vi "DRC Send Command_prev.vi"(2 "StringInput":string, 3 "Input":dbl min=0.0 format="%.3f", 4 "Command":T1(ring), 5 "GPIB Address":string) -> (0 "Output":dbl format="%.2f", 1 "Response":string)   [LabVIEW 2019]
panel:
  in  "CHANNEL":bool
  in  "CONTROLLER TYPE":bool
  out "error out":errorcluster
  in  "error in (no error)":errorcluster
  # "setpoint, heater value"
  # "temperature,etc."
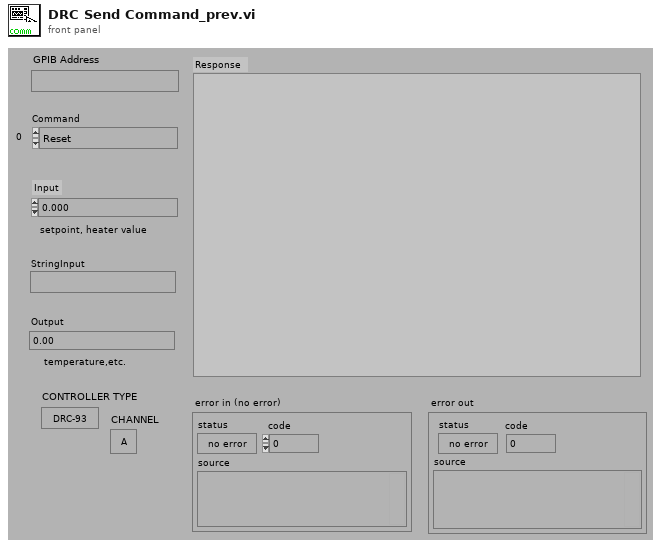
[diagram p1: front panel]
types:
  T1 = enum16{"Reset", "Raw_WriteRead", "ReadTemp", "ReadControl", "WriteSetPoint", "ReadSetPoint", "ManualHeatPwr", "HeaterOff", "SetHeaterScale", "SetProportional(gain)", "SetIntegrate(reset)", "SetDerivative(rate)", "SendCalibration", "ReadCalibration", "SelectCurve", "GetControlInfo", "Change units", "GetDCSP_Reading", "GetPIDR_Reading", "ZeroNonVol_Mem"}
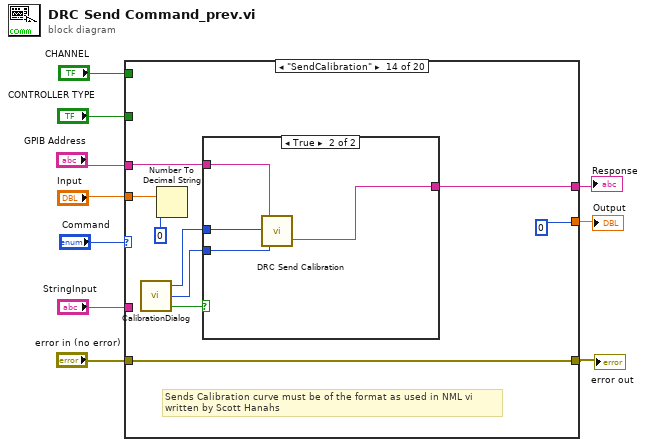
[diagram p0: block diagram]
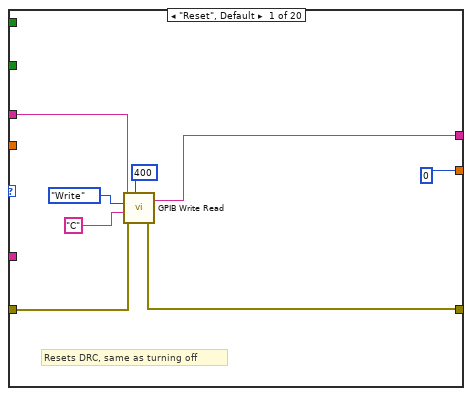
[diagram p2: hidden frame]
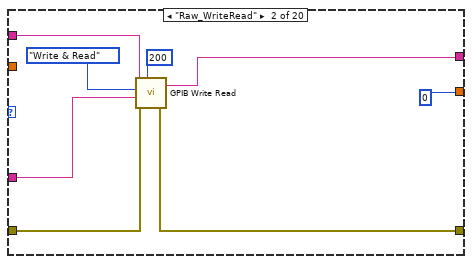
[diagram p3: hidden frame]
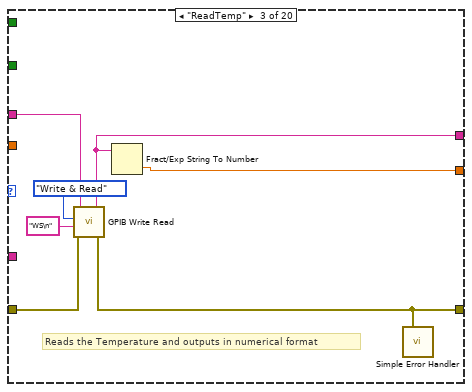
[diagram p4: hidden frame]
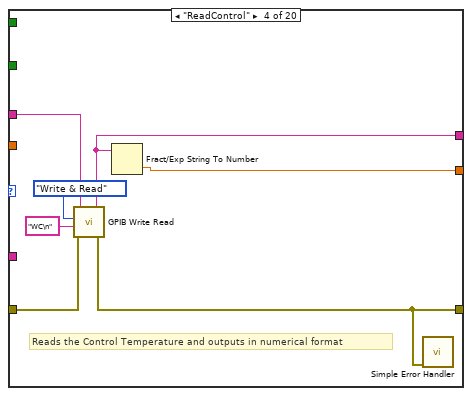
[diagram p5: hidden frame]
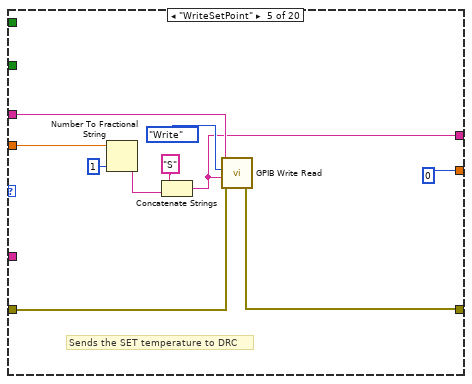
[diagram p6: hidden frame]
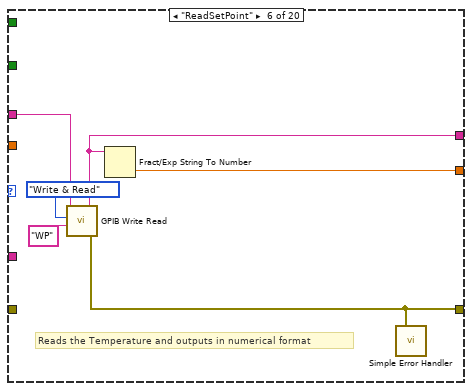
[diagram p7: hidden frame]
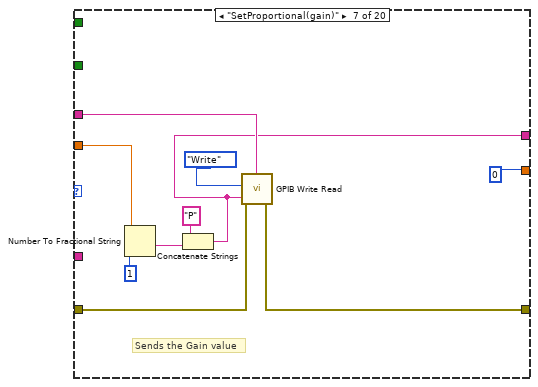
[diagram p8: hidden frame]
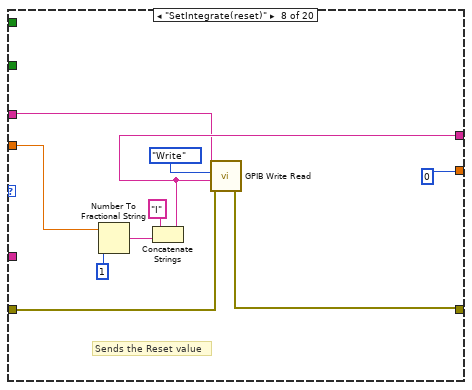
[diagram p9: hidden frame]
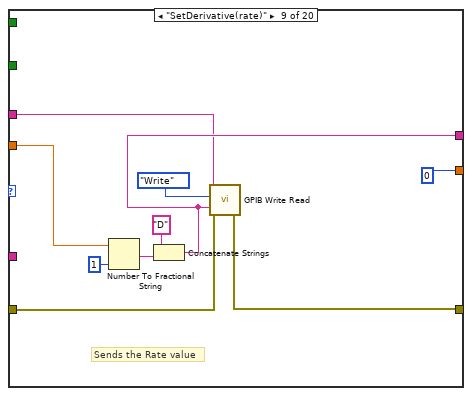
[diagram p10: hidden frame]
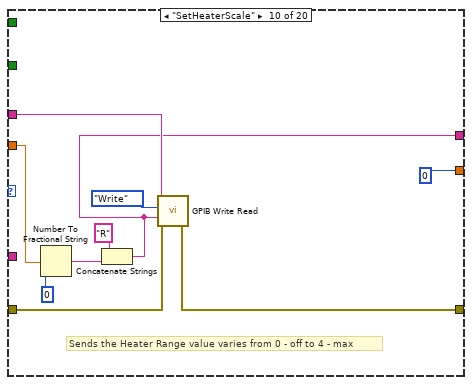
[diagram p11: hidden frame]
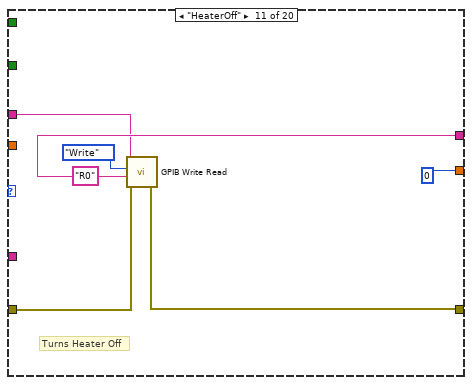
[diagram p12: hidden frame]
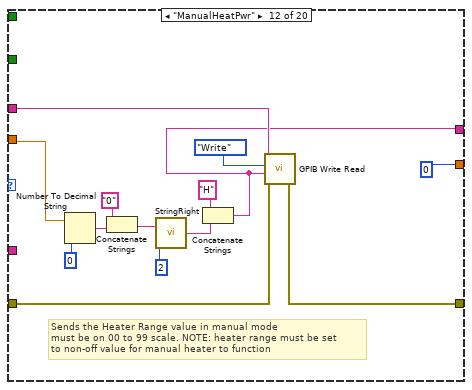
[diagram p13: hidden frame]
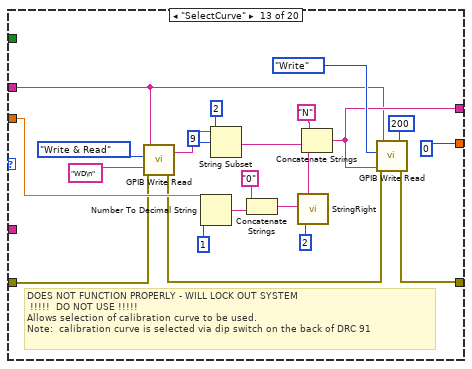
[diagram p14: hidden frame]
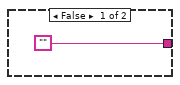
[diagram p15: hidden frame]
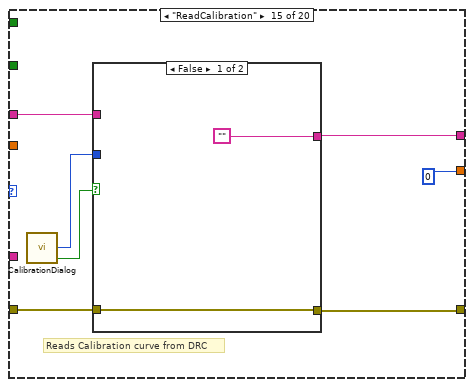
[diagram p16: hidden frame]
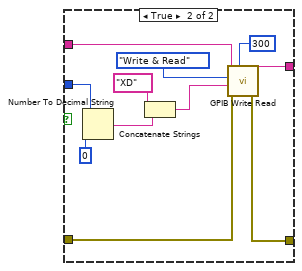
[diagram p17: hidden frame]
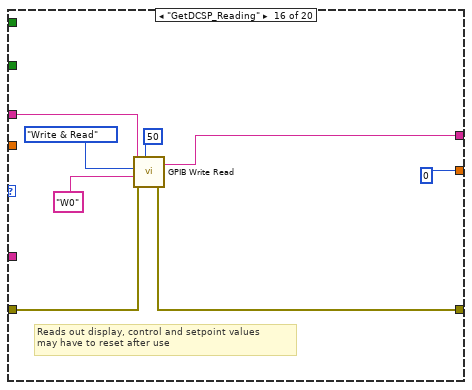
[diagram p18: hidden frame]
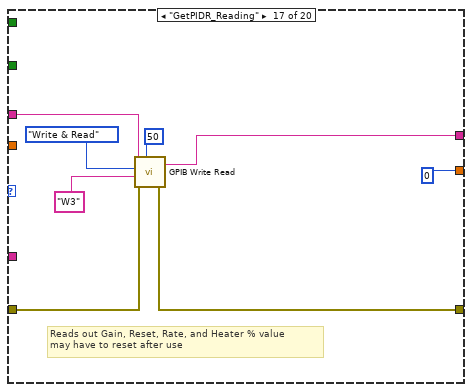
[diagram p19: hidden frame]
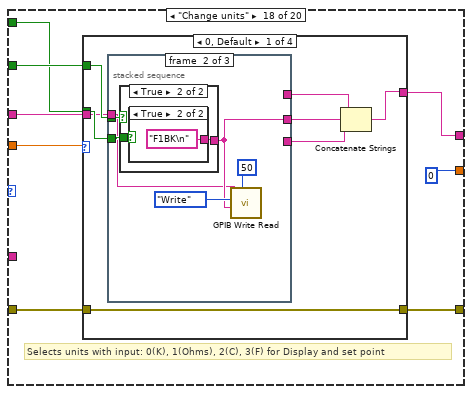
[diagram p20: hidden frame]
diagram:
  n1 = case shown="\"SendCalibration\"" "Command" {
    tunnel: [w15 w21 w30 w37 w41 w53 w59 w71 w81 w89 w101 w105 w124 w141 w155 w175 w182 w191 w336 "Non-Volatile memory has been reinitialized"] -> w10
    tunnel: "StringInput" -> [_ w20 _ _ _ _ _ _ _ _ _ _ _ _ _ _ _ _ _ _]
    tunnel: "Input" -> [_ _ _ _ w45 _ w63 w73 w83 w93 _ w114 w129 w143 _ _ _ w196 _ _]
    tunnel: "error in (no error)" -> [w17 w23 w33 w40 w44 _ w60 w69 w79 w90 w99 w106 w126 w140 w156 w177 w184 w195 w340 w347]
    tunnel: "CONTROLLER TYPE" -> [_ _ _ _ _ _ _ _ _ _ _ _ _ _ _ _ _ w194 w334 _]
    tunnel: "CHANNEL" -> [_ _ _ _ _ _ _ _ _ _ _ _ _ _ _ _ _ w193 _ _]
    tunnel: [w12 w22 w27 w34 w43 w51 w58 w68 w78 w88 w98 w104 w118 w140 w154 w176 w185 w192 w337 w345] -> w3
    tunnel: "GPIB Address" -> [w18 w24 w31 w38 w46 w56 w61 w70 w80 w91 w100 w107 w123 w147 w158 w178 w183 w190 w339 w348]
    tunnel: [0 0 w28 w35 0 w52 0 0 0 0 0 0 0 0 0 0 0 0 0 0] -> w1
    frame "Reset", Default {
      # "Resets DRC, same as turning off"
      n2 = call "GPIB Write Read.vi"("GPIB address"=w18, "Action"=enum16{"Write", "Read", "Write & Read"}."Write" ("y"), "String to Write"="C" ("InputString"), "error in (no error)"=w17, "wait (mS)"=400) -> ("String Read"=w15:string, "error out"=w12:errorcluster)
    }
    frame "Raw_WriteRead" {
      n3 = call "GPIB Write Read.vi"("GPIB address"=w24, "Action"=enum16{"Write", "Read", "Write & Read"}."Write & Read", "String to Write"=w20, "error in (no error)"=w23, "wait (mS)"=200) -> ("String Read"=w21:string, "error out"=w22:errorcluster)
    }
    frame "ReadTemp" {
      # "Reads the Temperature and outputs in numerical format"
      n4 = call "GPIB Write Read.vi"("GPIB address"=w31, "Action"=enum16{"Write", "Read", "Write & Read"}."Write & Read", "String to Write"="WS\n", "error in (no error)"=w33) -> ("String Read"=w30:string, "error out"=w27:errorcluster)  [unwired: 1 in]
      n5 = Fract/Exp String To Number(string=w30) -> (number=w28:dbl)  [unwired: 3 in, 1 out]
      n6 = call <vilib>:"Simple Error Handler.vi"("error in (no error)"=w27) -> ()  [unwired: 4 in, 5 out]
    }
    frame "ReadControl" {
      # "Reads the Control Temperature and outputs in numerical format"
      n7 = call "GPIB Write Read.vi"("GPIB address"=w38, "Action"=enum16{"Write", "Read", "Write & Read"}."Write & Read", "String to Write"="WC\n", "error in (no error)"=w40) -> ("String Read"=w37:string, "error out"=w34:errorcluster)  [unwired: 1 in]
      n8 = Fract/Exp String To Number(string=w37) -> (number=w35:dbl)  [unwired: 3 in, 1 out]
      n9 = call <vilib>:"Simple Error Handler.vi"("error in (no error)"=w34) -> ()  [unwired: 4 in, 5 out]
    }
    frame "WriteSetPoint" {
      # "Sends the SET temperature to DRC"
      n10 = Number To Fractional String(number=w45, precision (6)=i16 1) -> (F-format string=w49:string)  [unwired: 2 in]
      n11 = Concatenate Strings("S", w49) -> (w41:string)
      n12 = call "GPIB Write Read.vi"("GPIB address"=w46, "Action"=enum16{"Write", "Read", "Write & Read"}."Write" ("y"), "String to Write"=w41, "error in (no error)"=w44) -> ("error out"=w43:errorcluster)  [unwired: 1 in, 1 out]
    }
    frame "ReadSetPoint" {
      # "Reads the Temperature and outputs in numerical format"
      n13 = call "GPIB Write Read.vi"("GPIB address"=w56, "Action"=enum16{"Write", "Read", "Write & Read"}."Write & Read", "String to Write"="WP") -> ("String Read"=w53:string, "error out"=w51:errorcluster)  [unwired: 2 in]
      n14 = Fract/Exp String To Number(string=w53) -> (number=w52:dbl)  [unwired: 3 in, 1 out]
      n15 = call <vilib>:"Simple Error Handler.vi"("error in (no error)"=w51) -> ()  [unwired: 4 in, 5 out]
    }
    frame "SetProportional(gain)" {
      # "Sends the Gain value"
      n16 = Number To Fractional String(number=w63, precision (6)=i16 1) -> (F-format string=w65:string)  [unwired: 2 in]
      n17 = Concatenate Strings("P", w65) -> (w59:string)
      n18 = call "GPIB Write Read.vi"("GPIB address"=w61, "Action"=enum16{"Write", "Read", "Write & Read"}."Write" ("y"), "String to Write"=w59, "error in (no error)"=w60) -> ("error out"=w58:errorcluster)  [unwired: 1 in, 1 out]
    }
    frame "SetIntegrate(reset)" {
      # "Sends the Reset value"
      n19 = Number To Fractional String(number=w73, precision (6)=i16 1) -> (F-format string=w75:string)  [unwired: 2 in]
      n20 = Concatenate Strings("I", w75) -> (w71:string)
      n21 = call "GPIB Write Read.vi"("GPIB address"=w70, "Action"=enum16{"Write", "Read", "Write & Read"}."Write" ("y"), "String to Write"=w71, "error in (no error)"=w69) -> ("error out"=w68:errorcluster)  [unwired: 1 in, 1 out]
    }
    frame "SetDerivative(rate)" {
      # "Sends the Rate value"
      n22 = Number To Fractional String(number=w83, precision (6)=i16 1) -> (F-format string=w85:string)  [unwired: 2 in]
      n23 = Concatenate Strings("D", w85) -> (w81:string)
      n24 = call "GPIB Write Read.vi"("GPIB address"=w80, "Action"=enum16{"Write", "Read", "Write & Read"}."Write" ("y"), "String to Write"=w81, "error in (no error)"=w79) -> ("error out"=w78:errorcluster)  [unwired: 1 in, 1 out]
    }
    frame "SetHeaterScale" {
      # "Sends the Heater Range value varies from 0 - off to 4 - max"
      n25 = Number To Fractional String(number=w93, precision (6)=i16 0) -> (F-format string=w95:string)  [unwired: 2 in]
      n26 = Concatenate Strings("R", w95) -> (w89:string)
      n27 = call "GPIB Write Read.vi"("GPIB address"=w91, "Action"=enum16{"Write", "Read", "Write & Read"}."Write" ("y"), "String to Write"=w89, "error in (no error)"=w90) -> ("error out"=w88:errorcluster)  [unwired: 1 in, 1 out]
    }
    frame "HeaterOff" {
      w101 = "R0"
      # "Turns Heater Off"
      n28 = call "GPIB Write Read.vi"("GPIB address"=w100, "Action"=enum16{"Write", "Read", "Write & Read"}."Write" ("y"), "String to Write"=w101, "error in (no error)"=w99) -> ("error out"=w98:errorcluster)  [unwired: 1 in, 1 out]
    }
    frame "ManualHeatPwr" {
      # "Sends the Heater Range value in manual mode \nmust be on 00 to 99 scale. NOTE: heater range must be set \nto non-off value for manual heater to function"
      n29 = Number To Decimal String(number=w114, width (-)=i16 0 ("precision (6)")) -> (decimal integer string=w110:string)
      n30 = Concatenate Strings("0" ("Substring"), w110) -> (w112:string)
      n31 = call "StringRight.vi"("#chars"=2, "input string"=w112) -> ("output string"=w109:string)  [unwired: 1 in]
      n32 = Concatenate Strings("H", w109) -> (w105:string)
      n33 = call "GPIB Write Read.vi"("GPIB address"=w107, "Action"=enum16{"Write", "Read", "Write & Read"}."Write" ("y"), "String to Write"=w105, "error in (no error)"=w106) -> ("error out"=w104:errorcluster)  [unwired: 1 in, 1 out]
    }
    frame "SelectCurve" {
      # "DOES NOT FUNCTION PROPERLY - WILL LOCK OUT SYSTEM\n !!!!!  DO NOT USE !!!!! \nAllows selection of calibration curve to be used.\nNote:  calibration curve is selected via dip switch on the back of DRC 91"
      n34 = call "GPIB Write Read.vi"("GPIB address"=w123, "Action"=enum16{"Write", "Read", "Write & Read"}."Write & Read", "String to Write"="WD\n", "error in (no error)"=w126) -> ("String Read"=w122:string, "error out"=w121:errorcluster)  [unwired: 1 in]
      n35 = Number To Decimal String(number=w129, width (-)=i16 1 ("precision (6)")) -> (decimal integer string=w128:string)
      n36 = String Subset(string=w122, offset (0)=9, length (rest)=2 ("length")) -> (substring=w133:string)
      n37 = Concatenate Strings("0" ("Substring"), w128) -> (w135:string)
      n38 = call "StringRight.vi"("#chars"=2, "input string"=w135) -> ("output string"=w132:string)  [unwired: 1 in]
      n39 = Concatenate Strings("N" ("Substring"), w133, w132) -> (w124:string)
      n40 = call "GPIB Write Read.vi"("GPIB address"=w123, "Action"=enum16{"Write", "Read", "Write & Read"}."Write" ("y"), "String to Write"=w124, "error in (no error)"=w121, "wait (mS)"=200 ("length")) -> ("error out"=w118:errorcluster)  [unwired: 1 out]
    }
    frame "SendCalibration" {
      # "Sends Calibration curve must be of the format as used in NML vi\nwritten by Scott Hanahs"
      n41 = call "CalibrationDialog.vi"() -> ("OK 2"=w146:bool, "Curve Number"=w145:i32, "Sensor Type display"=w142:i32)
      n42 = Number To Decimal String(number=w143, width (-)=i16 0 ("precision (6)")) -> ()  [unwired: 1 out]
      n43 = case shown="True" w146 {
        tunnel: w147 -> [_ w150]
        tunnel: w145 -> [_ w152]
        tunnel: w142 -> [_ w151]
        tunnel: ["" w149] -> w141
        frame False {
        }
        frame True {
          n44 = call "DRC Send Calibration.vi"("Calibration #"=w152, "Sensor Type"=w151, "GPIB Address (VISA)"=w150) -> ("Curve Table for this Calibration"=w149:string)  [unwired: 1 out]
        }
      }
    }
    frame "ReadCalibration" {
      # "Reads Calibration curve from DRC"
      n45 = call "CalibrationDialog.vi"() -> ("OK 2"=w159:bool, "Curve Number"=w157:i32)  [unwired: 1 out]
      n46 = case shown="False" w159 {
        tunnel: w158 -> [_ w168]
        tunnel: w157 -> [_ w166]
        tunnel: w156 -> [w161 w164]
        tunnel: [w161 w163] -> w154
        tunnel: ["" w162] -> w155
        frame False {
        }
        frame True {
          n47 = Number To Decimal String(number=w166, width (-)=i16 0 ("precision (6)")) -> (decimal integer string=w165:string)
          n48 = Concatenate Strings("XD", w165) -> (w171:string)
          n49 = call "GPIB Write Read.vi"("GPIB address"=w168, "Action"=enum16{"Write", "Read", "Write & Read"}."Write & Read", "String to Write"=w171, "error in (no error)"=w164, "wait (mS)"=i16 300 ("precision (6)")) -> ("String Read"=w162:string, "error out"=w163:errorcluster)
        }
      }
    }
    frame "GetDCSP_Reading" {
      # "Reads out display, control and setpoint values\nmay have to reset after use"
      n50 = call "GPIB Write Read.vi"("GPIB address"=w178, "Action"=enum16{"Write", "Read", "Write & Read"}."Write & Read", "String to Write"="W0", "error in (no error)"=w177, "wait (mS)"=50) -> ("String Read"=w175:string, "error out"=w176:errorcluster)
    }
    frame "GetPIDR_Reading" {
      # "Reads out Gain, Reset, Rate, and Heater % value\nmay have to reset after use"
      n51 = call "GPIB Write Read.vi"("GPIB address"=w183, "Action"=enum16{"Write", "Read", "Write & Read"}."Write & Read", "String to Write"="W3", "error in (no error)"=w184, "wait (mS)"=50) -> ("String Read"=w182:string, "error out"=w185:errorcluster)
    }
    frame "Change units" {
      # "Selects units with input: 0(K), 1(Ohms), 2(C), 3(F) for Display and set point"
      n52 = case shown="0, Default" w196 {
        tunnel: w195 -> [w202 w237 w269 w304]
        tunnel: w194 -> [w204 w236 w272 w302]
        tunnel: w193 -> [w203 w235 w268 w303]
        tunnel: [w202 w237 w269 w304] -> w192
        tunnel: [w200 w234 w270 w305] -> w191
        tunnel: w190 -> [w197 w231 w265 w299]
        frame 0, Default {
          n53 = stacked-sequence {
            tunnel: w204 -> [_ w212 w222]
            tunnel: w203 -> [_ w211 w221]
            tunnel: [w206 _ _] -> w201
            tunnel: [_ w210 _] -> w199
            tunnel: [_ _ w223] -> w198
            tunnel: w197 -> [w205 w209 w220]
            frame #0 {
              w206 = "F0K\n"
              n54 = call "GPIB Write Read.vi"("GPIB address"=w205, "Action"=enum16{"Write", "Read", "Write & Read"}."Write" ("y"), "String to Write"=w206, "wait (mS)"=50) -> ()  [unwired: 1 in, 2 out]
            }
            frame #1 {
              n55 = case shown="True" w212 {
                tunnel: ["F1K\n" w217] -> w210
                tunnel: w211 -> [_ w216]
                frame False {
                }
                frame True {
                  n56 = case shown="True" w216 {
                    tunnel: ["F1AK\n" "F1BK\n"] -> w217
                    frame False {
                    }
                    frame True {
                    }
                  }
                }
              }
              n57 = call "GPIB Write Read.vi"("GPIB address"=w209, "Action"=enum16{"Write", "Read", "Write & Read"}."Write" ("y"), "String to Write"=w210, "wait (mS)"=50) -> ()  [unwired: 1 in, 2 out]
            }
            frame #2 {
              n58 = case shown="True" w222 {
                tunnel: ["" w228] -> w223
                tunnel: w221 -> [_ w227]
                frame False {
                }
                frame True {
                  n59 = case shown="False" w227 {
                    tunnel: ["F2AK\n" "F2BK\n"] -> w228
                    frame False {
                    }
                    frame True {
                    }
                  }
                }
              }
              n60 = call "GPIB Write Read.vi"("GPIB address"=w220, "Action"=enum16{"Write", "Read", "Write & Read"}."Write" ("y"), "String to Write"=w223, "wait (mS)"=50) -> ()  [unwired: 1 in, 2 out]
            }
          }
          n61 = Concatenate Strings(w201, w199, w198) -> (w200:string)
        }
        frame 1 {
          n62 = stacked-sequence {
            tunnel: w236 -> [_ w246 w257]
            tunnel: w235 -> [_ w245 w256]
            tunnel: [w240 _ _] -> w238
            tunnel: [_ _ w255] -> w232
            tunnel: [_ w244 _] -> w233
            tunnel: w231 -> [w239 w243 w254]
            frame #0 {
              w240 = "F0S\n"
              n63 = call "GPIB Write Read.vi"("GPIB address"=w239, "Action"=enum16{"Write", "Read", "Write & Read"}."Write" ("y"), "String to Write"=w240, "wait (mS)"=50) -> ()  [unwired: 1 in, 2 out]
            }
            frame #1 {
              n64 = case shown="True" w246 {
                tunnel: ["F1S\n" w251] -> w244
                tunnel: w245 -> [_ w250]
                frame False {
                }
                frame True {
                  n65 = case shown="True" w250 {
                    tunnel: ["F1AS\n" "F1BS\n"] -> w251
                    frame False {
                    }
                    frame True {
                    }
                  }
                }
              }
              n66 = call "GPIB Write Read.vi"("GPIB address"=w243, "Action"=enum16{"Write", "Read", "Write & Read"}."Write" ("y"), "String to Write"=w244, "wait (mS)"=50) -> ()  [unwired: 1 in, 2 out]
            }
            frame #2 {
              n67 = case shown="True" w257 {
                tunnel: ["" w262] -> w255
                tunnel: w256 -> [_ w261]
                frame False {
                }
                frame True {
                  n68 = case shown="False" w261 {
                    tunnel: ["F2AS\n" "F2BS\n"] -> w262
                    frame False {
                    }
                    frame True {
                    }
                  }
                }
              }
              n69 = call "GPIB Write Read.vi"("GPIB address"=w254, "Action"=enum16{"Write", "Read", "Write & Read"}."Write" ("y"), "String to Write"=w255, "wait (mS)"=50) -> ()  [unwired: 1 in, 2 out]
            }
          }
          n70 = Concatenate Strings(w238, w233, w232) -> (w234:string)
        }
        frame 2 {
          n71 = stacked-sequence {
            tunnel: w272 -> [_ w280 w291]
            tunnel: w268 -> [_ w279 w290]
            tunnel: [w274 _ _] -> w271
            tunnel: [_ _ w289] -> w267
            tunnel: [_ w278 _] -> w266
            tunnel: w265 -> [w273 w277 w288]
            frame #0 {
              w274 = "F0C\n"
              n72 = call "GPIB Write Read.vi"("GPIB address"=w273, "Action"=enum16{"Write", "Read", "Write & Read"}."Write" ("y"), "String to Write"=w274, "wait (mS)"=50) -> ()  [unwired: 1 in, 2 out]
            }
            frame #1 {
              n73 = case shown="False" w280 {
                tunnel: ["F1C\n" w285] -> w278
                tunnel: w279 -> [_ w284]
                frame False {
                }
                frame True {
                  n74 = case shown="False" w284 {
                    tunnel: ["F1AC\n" "F1BC\n"] -> w285
                    frame False {
                    }
                    frame True {
                    }
                  }
                }
              }
              n75 = call "GPIB Write Read.vi"("GPIB address"=w277, "Action"=enum16{"Write", "Read", "Write & Read"}."Write" ("y"), "String to Write"=w278, "wait (mS)"=50) -> ()  [unwired: 1 in, 2 out]
            }
            frame #2 {
              n76 = case shown="True" w291 {
                tunnel: ["" w296] -> w289
                tunnel: w290 -> [_ w295]
                frame False {
                }
                frame True {
                  n77 = case shown="True" w295 {
                    tunnel: ["F2AC\n" "F2BC\n"] -> w296
                    frame False {
                    }
                    frame True {
                    }
                  }
                }
              }
              n78 = call "GPIB Write Read.vi"("GPIB address"=w288, "Action"=enum16{"Write", "Read", "Write & Read"}."Write" ("y"), "String to Write"=w289, "wait (mS)"=50) -> ()  [unwired: 1 in, 2 out]
            }
          }
          n79 = Concatenate Strings(w271, w266, w267) -> (w270:string)
        }
        frame 3 {
          n80 = stacked-sequence {
            tunnel: w302 -> [_ w314 w325]
            tunnel: w303 -> [_ w313 w324]
            tunnel: [w308 _ _] -> w306
            tunnel: [_ _ w323] -> w301
            tunnel: [_ w312 _] -> w300
            tunnel: w299 -> [w307 w311 w322]
            frame #0 {
              w308 = "F0F\n"
              n81 = call "GPIB Write Read.vi"("GPIB address"=w307, "Action"=enum16{"Write", "Read", "Write & Read"}."Write" ("y"), "String to Write"=w308, "wait (mS)"=50) -> ()  [unwired: 1 in, 2 out]
            }
            frame #1 {
              n82 = case shown="False" w314 {
                tunnel: ["F1F\n" w319] -> w312
                tunnel: w313 -> [_ w318]
                frame False {
                }
                frame True {
                  n83 = case shown="False" w318 {
                    tunnel: ["F1AF\n" "F1BF\n"] -> w319
                    frame False {
                    }
                    frame True {
                    }
                  }
                }
              }
              n84 = call "GPIB Write Read.vi"("GPIB address"=w311, "Action"=enum16{"Write", "Read", "Write & Read"}."Write" ("y"), "String to Write"=w312, "wait (mS)"=50) -> ()  [unwired: 1 in, 2 out]
            }
            frame #2 {
              n85 = case shown="True" w325 {
                tunnel: ["" w330] -> w323
                tunnel: w324 -> [_ w329]
                frame False {
                }
                frame True {
                  n86 = case shown="True" w329 {
                    tunnel: ["F2AF\n" "F2BF\n"] -> w330
                    frame False {
                    }
                    frame True {
                    }
                  }
                }
              }
              n87 = call "GPIB Write Read.vi"("GPIB address"=w322, "Action"=enum16{"Write", "Read", "Write & Read"}."Write" ("y"), "String to Write"=w323, "wait (mS)"=50) -> ()  [unwired: 1 in, 2 out]
            }
          }
          n88 = Concatenate Strings(w306, w300, w301) -> (w305:string)
        }
      }
    }
    frame "GetControlInfo" {
      # "Reads out sample, control and A and B input information\nmay have to reset after use"
      n89 = case shown="False" w334 {
        tunnel: ["WD\n" "W1\n"] -> w335
        frame False {
        }
        frame True {
        }
      }
      n90 = call "GPIB Write Read.vi"("GPIB address"=w339, "Action"=enum16{"Write", "Read", "Write & Read"}."Write & Read", "String to Write"=w335, "error in (no error)"=w340) -> ("String Read"=w336:string, "error out"=w337:errorcluster)  [unwired: 1 in]
    }
    frame "ZeroNonVol_Mem" {
      n91 = call "GPIB Write Read.vi"("GPIB address"=w348, "Action"=enum16{"Write", "Read", "Write & Read"}."Write", "String to Write"="XR&I*XR&I*XR&I*XR&I*XR&I*", "error in (no error)"=w347) -> ("error out"=w345:errorcluster)  [unwired: 1 in, 1 out]
    }
  }
  "Response" <- w10
  "error out" <- w3
  "Output" <- w1
